vi "get load fw progress.vi"(8 "error in (no error)":errorcluster, 11 "progress":dbl) -> (0 "error out":errorcluster, 2 "function return":bool, 3 "progress out":dbl)   [LabVIEW 2015, in "XGL_DPP.lvlib"]
doc: "EXTERN DECLSPEC bool CALL_CONV get_load_fw_progress(double * progress);"
uses:
  XGL_DPP.lvlib
  XGL_DPP.dll
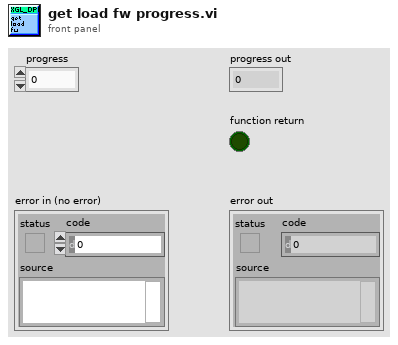
[diagram p1: front panel]
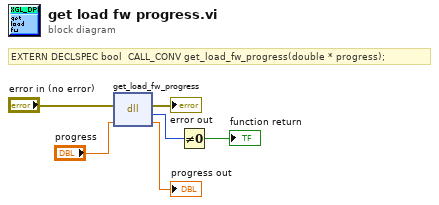
[diagram p0: block diagram]
diagram:
  # "EXTERN DECLSPEC bool  CALL_CONV get_load_fw_progress(double * progress);"
  n1 = dll-call lib="D:/Users/XRF/Desktop/Scanning Software_Demokritos_2015_v7/libs/Vis_2/XGL_DPP.*" fn="get_load_fw_progress"(error in="error in (no error)", "progress"="progress") -> (error out=→"error out":errorcluster, w5:u8, "progress"=→"progress out":dbl)  [unwired: 2 in, 1 out]
  n2 = Not Equal To 0?(x=w5) -> (x != 0?=→"function return":bool)
